vi "Subscribe.vi"(6 "Time out (ms)":i32=1000, 7 "Topic":string, 8 "error in (no error)":errorcluster, 9 "WAMP Client in":refnum<class "WAMP Client.lvclass">) -> (0 "Subscription ID":u32, 1 "Success?":bool, 2 "error out":errorcluster, 3 "WAMP Client out":refnum<class "WAMP Client.lvclass">)   [LabVIEW 2020, in "WAMP Client.lvclass"]
uses:
  <userlib>/lvwamp/WAMP Client/WAMP Client.lvclass
  <userlib>/lvwamp/WAMP Client/WAMP Client.lvclass/WAMP Client.ctl
  <userlib>/lvwamp/MessageCodes.ctl
  <vilib>/ErrorRing/Error Ring.xnode
  <vilib>/Utility/error.llb/Error Cluster From Error Code.vi
  <vilib>/numeric/Random Number (Range) U64.vi
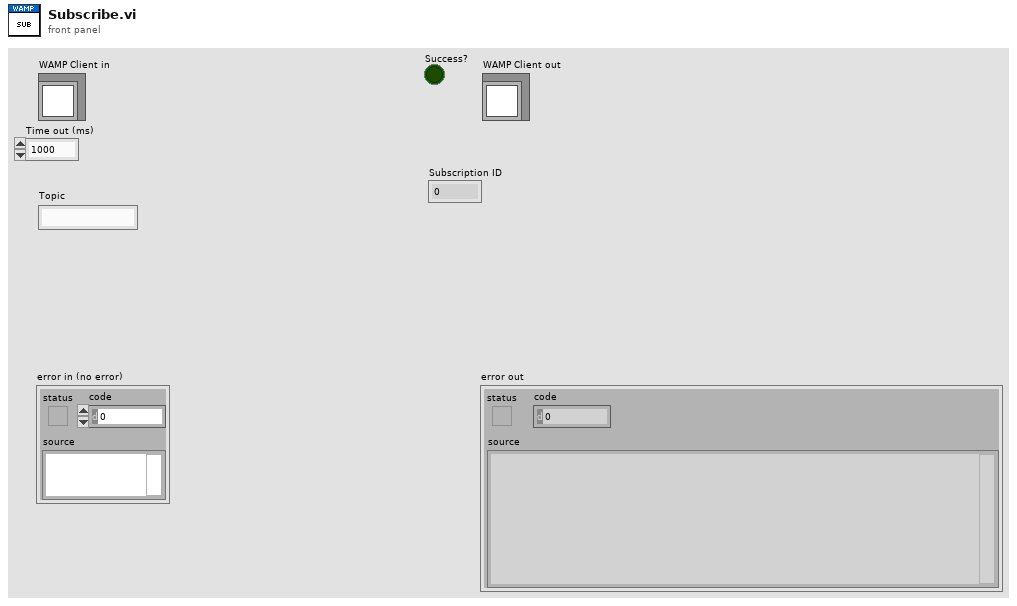
[diagram p1: front panel]
types:
  T1 = typedef "WAMP Client.lvclass/MessageCodes.ctl" = u16
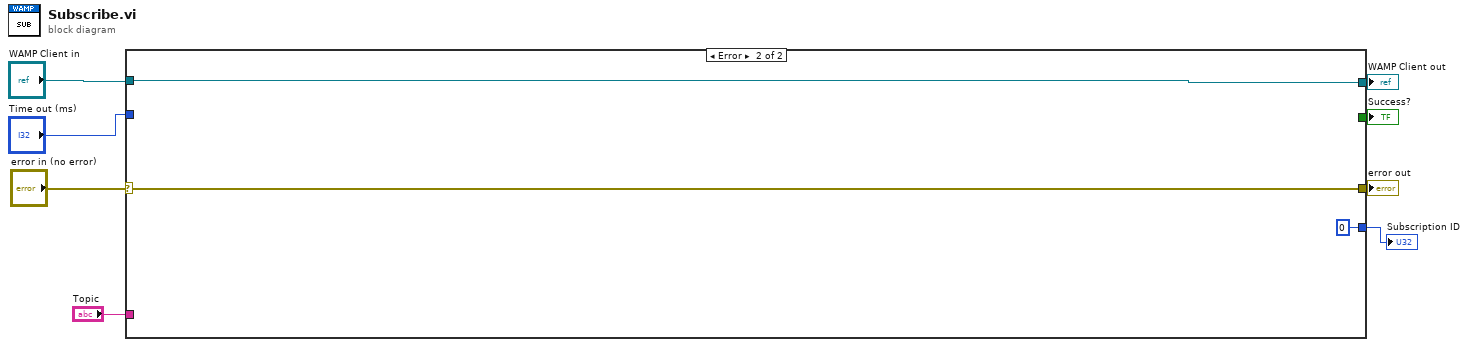
[diagram p0: block diagram]
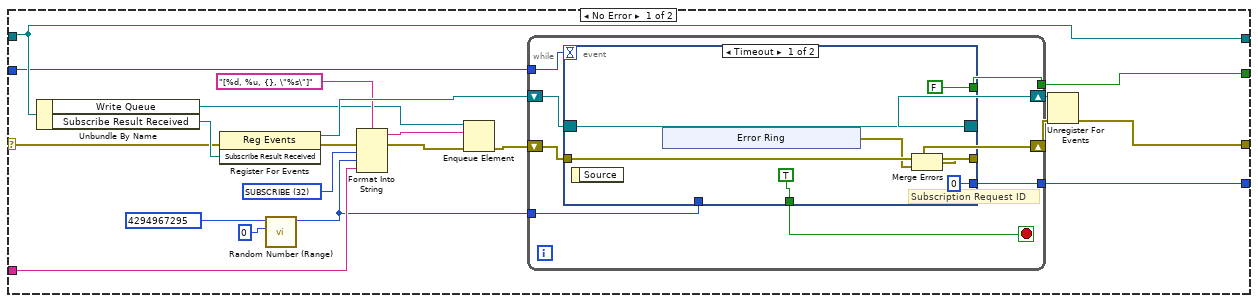
[diagram p2: hidden frame]
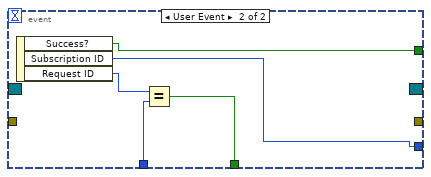
[diagram p3: hidden frame]
diagram:
  n1 = case shown="Error" "error in (no error)" {
    selector: "error in (no error)" -> [w14 w58]
    tunnel: [w12 w58] -> w7
    tunnel: [w17 w57] -> w5
    tunnel: "WAMP Client in" -> [w17 w57]
    tunnel: "Topic" -> [w29 _]
    tunnel: [w25 _] -> w3
    tunnel: "Time out (ms)" -> [w15 _]
    tunnel: [w9 u32 0 ("Subscription ID")] -> w1
    frame No Error {
      w20 = T1 32 items=["HELLO"=1, "WELCOME"=2, "ABORT"=3, "GOODBYE"=6, "ERROR"=8, "PUBLISH"=16, "PUBLISHED"=17, "SUBSCRIBE"=32, "SUBSCRIBED"=33, "UNSUBSCRIBE"=34, "UNSUBSCRIBED"=35, "EVENT"=36, "CALL"=48, "RESULT"=59, "REGISTER"=64, "REGISTERED"=65, "UNREGISTER"=66, "UNREGISTERED"=67, "INVOCATION"=68, "YIELD"=70] ("Message Codes")
      n2 = Unbundle By Name(w17) -> ("Write Queue"=w16:refnum<queue>, "Subscribe Result Received"=w24:refnum<user-event>)
      n3 = register-events(error in=w14, w24) -> (reference out=w26:refnum<event-registration>, error out=w19:errorcluster)  [unwired: 1 in]
      n4 = call-poly <vilib>:"Random Number (Range).vi"("lower bound (0)"=u32 0, "upper bound (100)"=u32 4294967295) -> ("number"=w10:u64)  [unwired: 9 in]
      n5 = Format Into String(format string="[%d, %u, {}, \"%s\"]" ("element"), error in=w19, w20, w10, w29) -> (resulting string=w22:string, error out=w23:errorcluster)  [unwired: 1 in]
      n6 = Enqueue Element(queue=w16, element=w22, error in (no error)=w23) -> (error out=w18:errorcluster)  [unwired: 1 in, 2 out]
      n7 = while {
        tunnel: [w37] -> w25
        tunnel: w15 -> [w31]
        shift-right: [w34] -> w11
        shift-left: w26 -> [w38]
        shift-right: [w35] -> w13
        shift-left: w18 -> [w36]
        tunnel: w10 -> [w33]
        tunnel: [w30] -> w9
        stop <- w32 stop-if-true
        # "Subscription Request ID"
        n8 = event shown="[0] Timeout" {
          selector: w38 -> [w41 _]
          dyn-events: [w41 _] -> w34
          timeout: w31 -> [_ _]
          tunnel: [FALSE ("Success?") w52] -> w37
          tunnel: [w42 _] -> w35
          tunnel: w36 -> [w44 _]
          tunnel: w33 -> [_ w54]
          tunnel: [TRUE w53] -> w32
          tunnel: [u32 0 ("Subscription ID") w51] -> w30
          event Timeout {
            n9 = event-data() -> ()  [unwired: 1 in, 1 out]
            n10 = xnode "Error Ring"() -> ("error out"=w43:errorcluster)
            n11 = Merge Errors(w44, w43) -> (w42:errorcluster)
          }
          event User Event {
            n12 = event-data() -> ("Success?"=w52:bool, "Subscription ID"=w51:u32, "Request ID"=w55:u32)  [unwired: 1 in]
            n13 = Equal?(x=w55, y=w54) -> (x = y?=w53:bool)
          }
        }
      }
      n14 = Unregister For Events(event registration refnum=w11, error in=w13) -> (error out=w12:errorcluster)
    }
    frame Error {
    }
  }
  "error out" <- w7
  "WAMP Client out" <- w5
  "Success?" <- w3
  "Subscription ID" <- w1
